vi "Add Element in Array Altitude Observers.vi"(8 "error in (no error)":errorcluster, 10 "Observer input":refnum<class "Observer.lvclass">, 11 "Vessel in":refnum<class "Vessel.lvclass">) -> (0 "error out":errorcluster, 2 "Index":i32, 3 "Vessel out":refnum<class "Vessel.lvclass">)   [LabVIEW 2014, in "Vessel.lvclass"]
uses:
  Vessel.lvclass
  Observer/Observer.lvclass
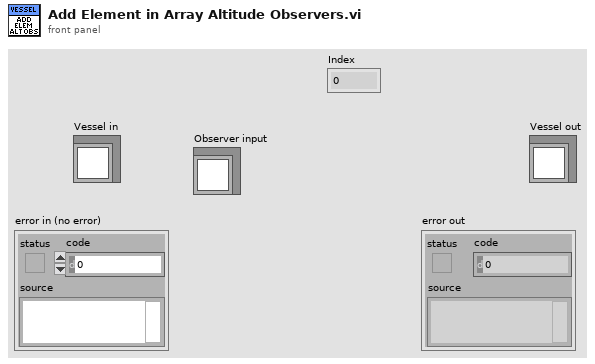
[diagram p1: front panel]
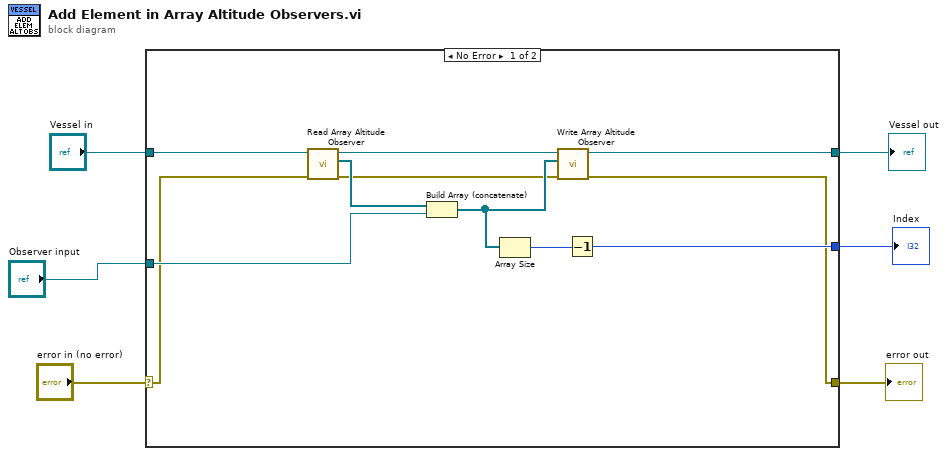
[diagram p0: block diagram]
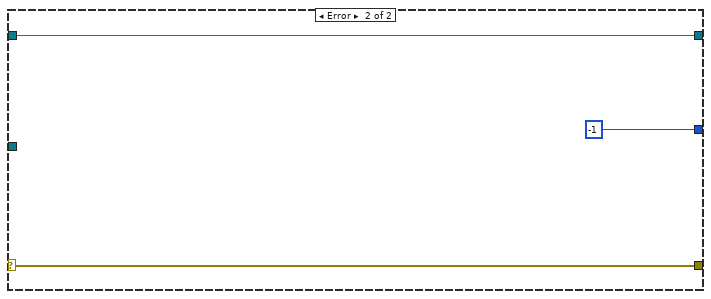
[diagram p2: hidden frame]
diagram:
  n1 = case shown="No Error" "error in (no error)" {
    selector: "error in (no error)" -> [w12 w20]
    tunnel: [w10 w20] -> w5
    tunnel: [w11 w19] -> w4
    tunnel: "Vessel in" -> [w14 w19]
    tunnel: "Observer input" -> [w17 _]
    tunnel: [w15 -1] -> w1
    frame No Error {
      n2 = call-dynamic "Read Array Altitude Observer.vi"("error in (no error)"=w12, "Vessel in"=w14) -> ("error out"=w7:errorcluster, "Array Altitude Observer"=w13:refnum<class "Observer.lvclass">[], "Vessel out"=w8:refnum<class "Vessel.lvclass">)  [unwired: 7 in]
      n3 = Build Array (concatenate)(w13, w17) -> (w9:refnum<class "Observer.lvclass">[])
      n4 = Array Size(array=w9) -> (size(s)=w16:i32)
      n5 = call-dynamic "Write Array Altitude Observer.vi"("error in (no error)"=w7, "Array Altitude Observer"=w9, "Vessel in"=w8) -> ("error out"=w10:errorcluster, "Vessel out"=w11:refnum<class "Vessel.lvclass">)  [unwired: 7 in]
      n6 = Decrement(x=w16) -> (x-1=w15:i32)
    }
    frame Error {
    }
  }
  "error out" <- w5
  "Vessel out" <- w4
  "Index" <- w1
